vi "Set Initialization Data - sequenceManagerWkr.vi"(8 "error in":errorcluster, 11 "sequenceManagerTest in":refnum<class "sequenceManagerTest.lvclass">) -> (0 "error out":errorcluster, 3 "sequenceManagerTest out":refnum<class "sequenceManagerTest.lvclass">)   [LabVIEW 2023, in "sequenceManagerTest.lvclass"]
doc: "In this VI you can set the initialization data of a statically-linked subWorker."
uses:
  sequenceManagerTest.lvclass
  sequenceManagerTest.lvclass/sequenceManagerTest.ctl
  sequenceManagerWorker/Response Cases.ctl
  sequenceManagerWorker/sequenceManagerWorker.lvclass
  sequenceManagerWorker/Initialization Data.ctl
  C:/Program Files (x86)/National Instruments/LabVIEW 2023/vi.lib/addons/_Workers/Library/Classes/Worker/Worker.lvclass
  C:/Program Files (x86)/National Instruments/LabVIEW 2023/vi.lib/addons/_Workers/Library/Classes/Workers Object/Workers Object.lvclass
  C:/Cutiss/ZE_Easy.SequenceManager/LabViewWrapper/Easy.SequenceManager.Worker/Workers/sequenceManagerWorker/sequenceManagerWorker.lvclass
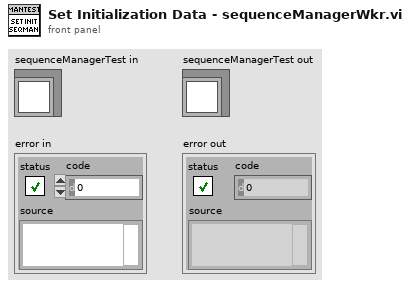
[diagram p1: front panel]
types:
  T1 = typedef "sequenceManagerWorker.lvclass/Initialization Data.ctl" = cluster{"Response Cases":T2}
  T2 = typedef "sequenceManagerWorker.lvclass/Response Cases.ctl" = cluster{"Placeholder - Can be deleted":string}
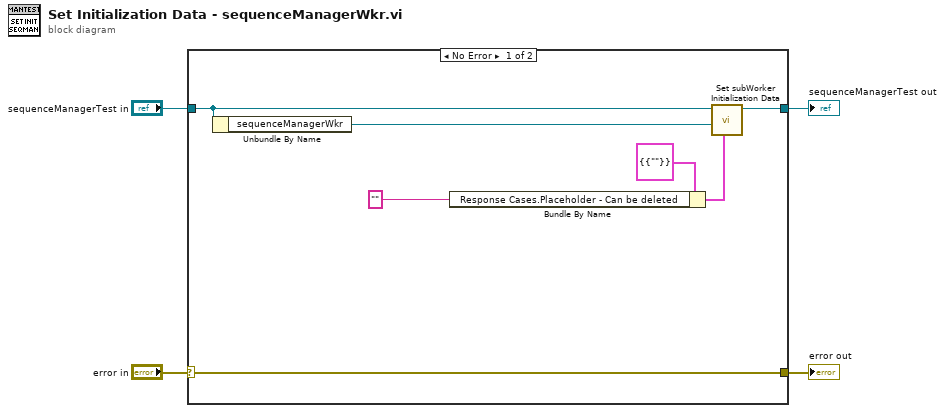
[diagram p0: block diagram]
diagram:
  n1 = case shown="No Error" "error in" {
    selector: "error in" -> [w11 w13]
    tunnel: [w11 w13] -> w3
    tunnel: [w9 w12] -> w2
    tunnel: "sequenceManagerTest in" -> [w8 w12]
    frame No Error {
      n2 = Unbundle By Name(w8) -> ("sequenceManagerWkr"=w10:refnum<class "sequenceManagerWorker.lvclass">)
      n3 = Bundle By Name(cluster=T1 {"Response Cases"={"Placeholder - Can be deleted"=""}} ("Initialization Data"), "Response Cases.Placeholder - Can be deleted"="" ("Placeholder")) -> (w6:T1)
      n4 = call-dynamic "Set subWorker Initialization Data.vi"("Initialization Data"=w6, "subWorker"=w10, "Worker"=w8) -> ("Worker out"=w9:refnum<class "sequenceManagerTest.lvclass">)  [unwired: 8 in]
    }
    frame Error {
    }
  }
  "error out" <- w3
  "sequenceManagerTest out" <- w2
